vi "GetInterfaceName.vi"(0 "reference in":refnum<class "G#Interface.lvclass">, 5 "error in (no error)":errorcluster) -> (14 "reference out":refnum<class "G#Interface.lvclass">, 15 "interface name":string, 16 "lvlib hierarchy":string[](array[string]), 17 "full interface name":string, 19 "error out":errorcluster)   [LabVIEW 2020, in "G#Interface.lvclass"]
doc: "Returns the class name, full class name , lvlib hierarchy for the specified object."
uses:
  G#Interface.lvclass
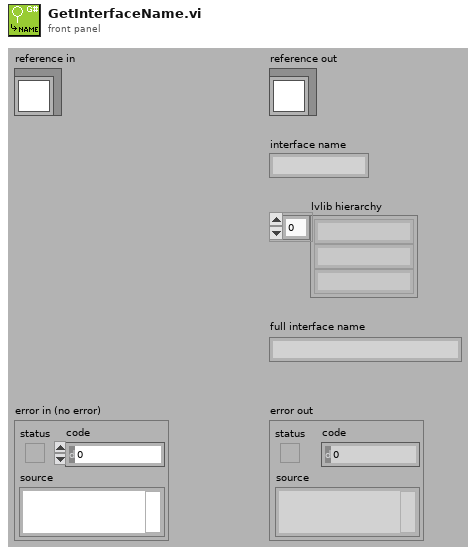
[diagram p1: front panel]
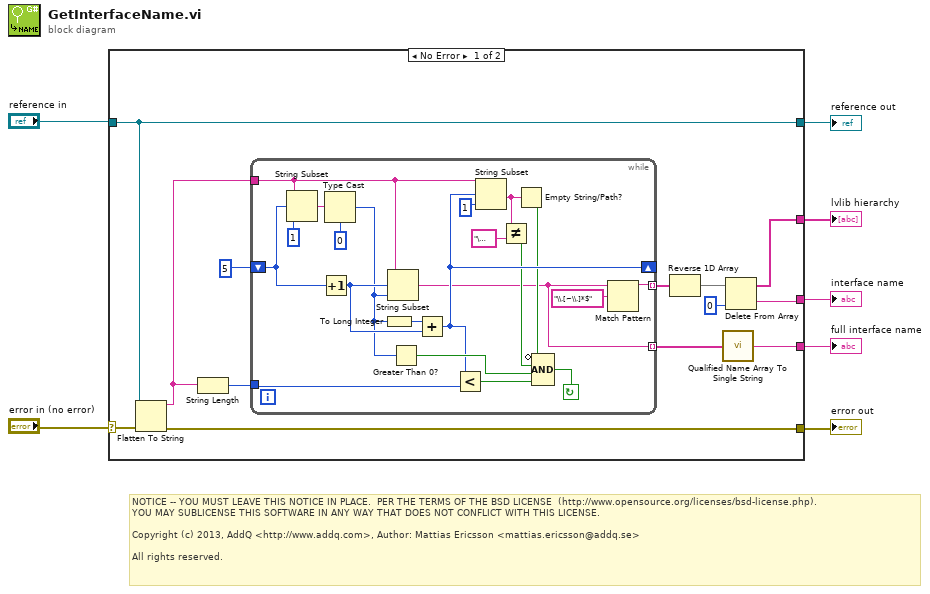
[diagram p0: block diagram]
diagram:
  # "NOTICE -- YOU MUST LEAVE THIS NOTICE IN PLACE.  PER THE TERMS OF THE BSD LICENSE  (http://www.opensource.org/licenses/bsd-license.php).\nYOU MAY SUBLICENSE THIS SOFTWARE IN ANY WAY THAT DOES NOT CONFLICT WITH THIS LICENSE.\n\nCopyright (c) 2013, AddQ <http://www.addq.com>, Author: Mattias Ericsson <mattias.ericsson@addq.se>\n\nAll rights reserved."
  n1 = case shown="No Error" "error in (no error)" {
    selector: "error in (no error)" -> [w19 w42]
    tunnel: "reference in" -> [w18 w43]
    tunnel: [w20 w42] -> w1
    tunnel: [w18 w43] -> w6
    tunnel: [w10 _] -> w5
    tunnel: [w11 _] -> w4
    tunnel: [w14 _] -> w3
    frame No Error {
      n2 = Flatten To String(anything=w18, error in (no error)=w19) -> (data string=w16:string, error out=w20:errorcluster)  [unwired: 2 in, 1 out]
      n3 = String Length(string=w16) -> (length=w15:i32)
      n4 = while {
        tunnel: w16 -> [w26]
        shift-right: [w30] -> _
        shift-left: 5 -> [w35]
        tunnel: w15 -> [w37]
        tunnel: [w22] -> w9 mode=indexing
        tunnel: [w21] -> w8 mode=indexing
        stop <- w36 continue-if-true
        n5 = String Subset(string=w26, offset (0)=w35, length (rest)=1 ("length (rest)")) -> (substring=w33:string)
        n6 = Increment(x=w35) -> (x+1=w41:i32)
        n7 = Type Cast(type=u8 0 ("default (0 U32)"), x=w33) -> (*(type *) &x=w31:u8)
        n8 = To Long Integer(number=w31) -> (32bit integer=w40:i32)
        n9 = String Subset(string=w26, offset (0)=w41, length (rest)=w31) -> (substring=w21:string)
        n10 = Greater Than 0?(x=w31) -> (x > 0?=w39:bool)
        n11 = Add(x=w40, y=w41) -> (x+y=w30:i32)
        n12 = Less?(x=w30, y=w37) -> (x < y?=w38:bool)
        n13 = String Subset(string=w26, offset (0)=w30, length (rest)=1 ("length (rest)")) -> (substring=w25:string)
        n14 = Not Equal?(x=w25, y="\u0000") -> (x != y?=w27:bool)
        n15 = Empty String/Path?(string/path=w25) -> (empty?=w24:bool)
        n16 = Compound Arithmetic op=AND(invert w24, w27, w39, w38) -> (w36:bool)
        n17 = Match Pattern(string=w21, regular expression="\\.[~\\.]*$") -> (before substring=w22:string)  [unwired: 4 out]
      }
      n18 = Reverse 1D Array(array=w9) -> (reversed array=w12:string[])
      n19 = call <vilib>:"Qualified Name Array To Single String.vi"("Fully Qualified Array"=w8) -> ("Fully Qualified String"=w14:string)
      n20 = Delete From Array(array=w12, index=0) -> (deleted portion=w11:string, array with subset deleted=w10:string[])  [unwired: 1 in]
    }
    frame Error {
    }
  }
  "reference out" <- w6
  "interface name" <- w4
  "lvlib hierarchy" <- w5
  "full interface name" <- w3
  "error out" <- w1
